vi "Notebook Main VI Name.vi"() -> ()   [LabVIEW 2019, in "Notebook.lvlib"]
uses:
  Notebook.lvlib
panel:
  in  "Main VI Name":string
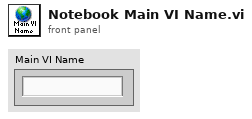
[diagram p1: front panel]
diagram:
